vi "FTW-SQLite-Core-PrepareStatement.vi"(0 "SQLite Connection":refnum<data-value>, 5 "SQL Statement":string, 11 "error in":errorcluster) -> (2 "Begin Timestamp":dbl format="%.3fmsec\n%<%D:%H:%M:%S%3u>t", 3 "Compile Time":dbl format="%.4psec", 4 "SQLite Connection out":refnum<data-value>, 6 "Library Filepath":path, 8 "Prepared Statements":i64[](array[numeric]) format="0x%016x", 15 "error out":errorcluster)   [LabVIEW 2015]
uses:
  FTW-SQLite-Core-Structure.ctl
panel:
  # "Inputs"
  # "Outputs"
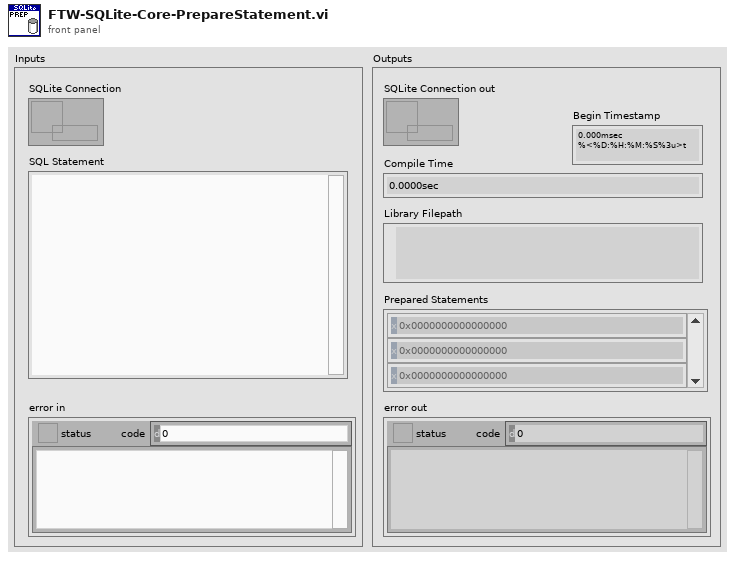
[diagram p1: front panel]
types:
  T1 = typedef "FTW-SQLite-Core-Structure.ctl" = cluster{"Connection":u64}
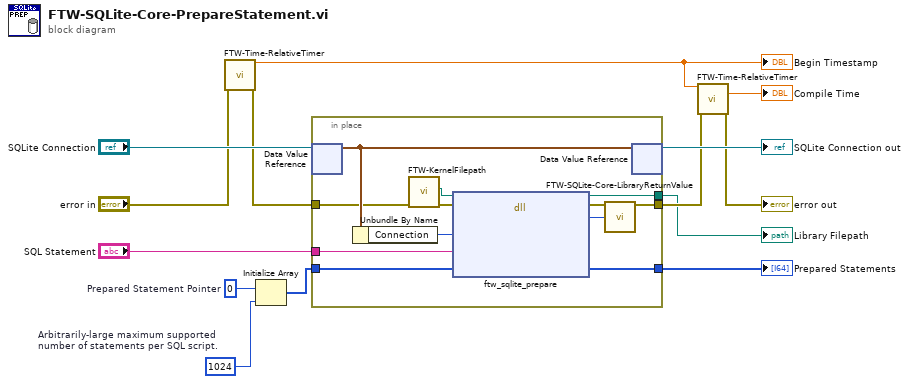
[diagram p0: block diagram]
diagram:
  w4 = 1024  # Arbitrarily-large maximum supported number of statements per SQL script.
  w3 = i64 0  # Prepared Statement Pointer
  n1 = call "FTW-Time-RelativeTimer.vi"("error in"="error in") -> ("Current Timer Value"=w5:dbl, "error out"=w9:errorcluster)  [unwired: 12 in, 1 out]
  "Begin Timestamp" <- w5
  n2 = Initialize Array(w3, w4) -> (w2:i64[])
  n3 = in-place {
    in-place-border: [w26] -> w8
    in-place-border: "SQL Statement" -> [w25]
    in-place-border: w9 -> [w17]
    in-place-border: [w20] -> w12
    in-place-border: w2 -> [w19]
    in-place-border: [w15] -> w1
    n4 = in-place-dvr #1("SQLite Connection") -> (w23:T1)  [unwired: 1 out]
    n5 = Unbundle By Name(w23) -> ("Connection"=w24:u64)
    n6 = call "FTW-KernelFilepath.vi"("error in"=w17) -> ("error out"=w16:errorcluster, "Library Filepath"=w18:path)  [unwired: 8 in, 1 out]
    n7 = dll-call lib="?" fn="ftw_sqlite_prepare"(path in=w18, error in=w16, "Connection Handle"=w24, "SQL Script"=w25, "Statements"=w19) -> (path out=w15:path, error out=w22:errorcluster, "Return Value"=w21:i32, "Statements"=w20:i64[])  [unwired: 3 in]
    n8 = call "FTW-SQLite-Core-LibraryReturnValue.vi"("error in"=w22, "Return Value"=w21) -> ("error out"=w26:errorcluster)  [unwired: 13 in]
    n9 = in-place-dvr #1(w23) -> (→"SQLite Connection out":refnum<data-value>)  [unwired: 1 out]
  }
  "Prepared Statements" <- w12
  "Library Filepath" <- w1
  n10 = call "FTW-Time-RelativeTimer.vi"("Previous Timer Value"=w5, "error in"=w8) -> ("Elapsed Time"=→"Compile Time":dbl, "error out"=→"error out":errorcluster)  [unwired: 11 in, 1 out]
